vi "Concatenate PDF Standalone - V2.vi"(0 "New File name":path, 7 "PDF Files  to concatenate [ ]":T6[](array[typedef]), 11 "error in (no error)":errorcluster, 12 "PDF Details":T2, 13 "Permissions":T1={"User Password"="", "Owner Password"="", "Printing"=enum."Allow Printing", "Allow Modify Contents"=FALSE, "Allow Copy"=FALSE, "Allow Modify Annotations"=TRUE, "Allow Fill In "=TRUE, "Allow Screen Readers"=FALSE, "Allow Assembly"=FALSE}) -> (6 "Pages dimensions [ ] OUT":T3[](array[typedef]) {"Page Size" items=["Custom", "LETTER", "NOTE", "LEGAL", "TABLOID", "EXECUTIVE", "POSTCARD", "A0", "A1", "A2", "A3", "A4", "A5", "A6", "A7", "A8", "A9", "A10", "B0", "B1", "B2", "B3", "B4", "B5", "B6", "B7", "B8", "B9", "B10", "ARCH_E", "ARCH_D", "ARCH_C", "ARCH_B", "ARCH_A", "FLSA", "FLSE", "HALFLETTER", "_11X17", "ID_1", "ID_2", "ID_3", "LEDGER", "CROWN_QUARTO", "LARGE_CROWN_QUARTO", "DEMY_QUARTO", "ROYAL_QUARTO", "CROWN_OCTAVO", "LARGE_CROWN_OCTAVO", "DEMY_OCTAVO", "ROYAL_OCTAVO", "SMALL_PAPERBACK", "PENGUIN_SMALL_PAPERBACK", "PENGUIN_LARGE_PAPERBACK"]}, 15 "error out":errorcluster)   [LabVIEW 2019, in "Exaprom PDF.lvlib"]
doc: "Standalone.\n\nVersion 1.0\nDeveloped by Jean-Marc Simard\nCopyright © 2012, Exaprom Inc.\nAll rights reserved.\nLicense: BSD\n\nWith iTextSharp Library\n(http://itextsharp.sourceforge.net)"
uses:
  Controls/Concatenate Controls/PDF file to concatenate.ctl
  Controls/Page Controls/Page dimensions.ctl
  Controls/Page Controls/Page Orientation.ctl
  Controls/Initialization Controls/PDF Details.ctl
  Controls/Initialization Controls/File Permission Parameters.ctl
  Controls/General Controls/Create or close.ctl
  Controls/Concatenate Controls/PDF File and position.ctl
  Controls/Concatenate Controls/PDF file source.ctl
  Exaprom PDF.lvlib
  Controls/Page Controls/Page size.ctl
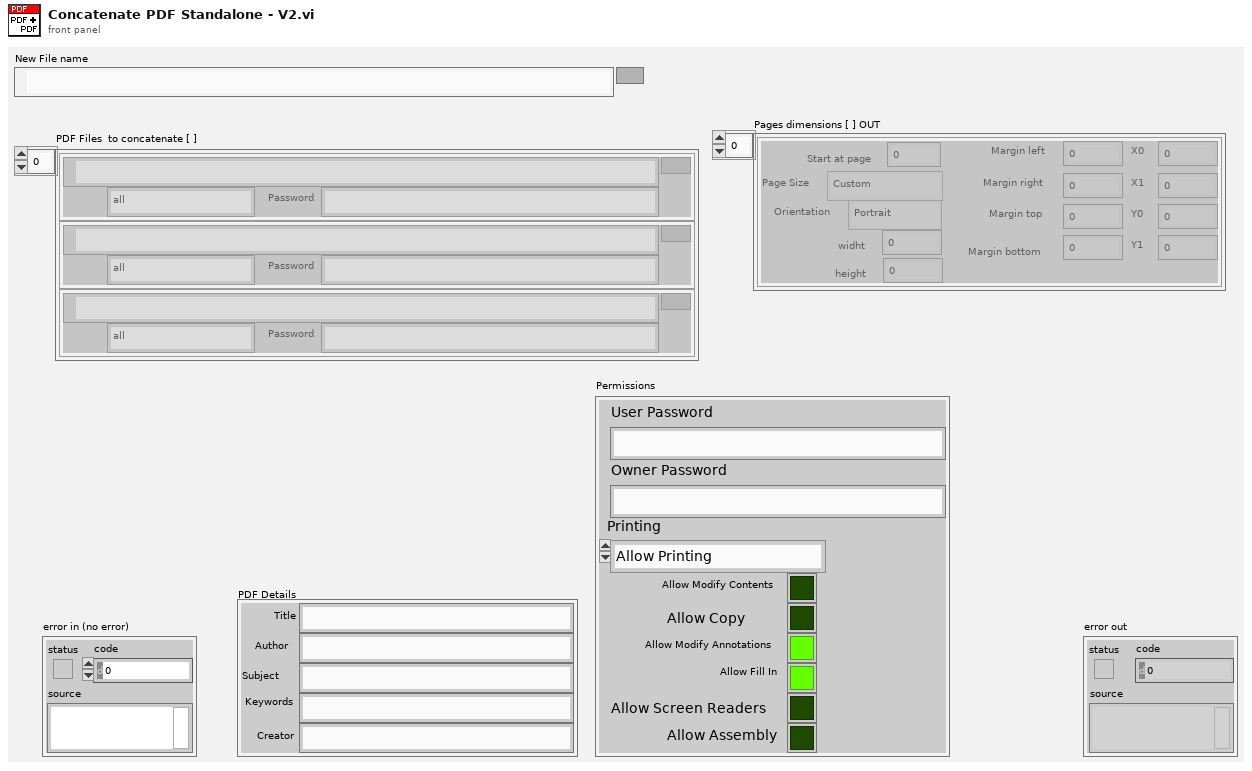
[diagram p1: front panel]
types:
  T1 = typedef "Exaprom PDF.lvlib/File Permission Parameters.ctl" = cluster{"User Password":string, "Owner Password":string, "Printing":enum16{"Allow Printing", "Allow Degraded Printing", "Don't Allow Printing"}, "Allow Modify Contents":bool, "Allow Copy":bool, "Allow Modify Annotations":bool, "Allow Fill In ":bool, "Allow Screen Readers":bool, "Allow Assembly":bool}
  T2 = typedef "Exaprom PDF.lvlib/PDF Details.ctl" = cluster{"Title":string, "Author":string, "Subject":string, "Keywords":string, "Creator":string}
  T3 = typedef "Exaprom PDF.lvlib/Page dimensions.ctl" = cluster{"Start at page":i32, "Page Size":T4, "Orientation":T5, "widht":sgl, "height":sgl, "Margin left":sgl, "Margin right":sgl, "Margin top":sgl, "Margin bottom":sgl, "X0":sgl, "X1":sgl, "Y0":sgl, "Y1":sgl}
  T4 = typedef "Exaprom PDF.lvlib/Page size.ctl" = i32
  T5 = typedef "Exaprom PDF.lvlib/Page Orientation.ctl" = enum16{"Portrait", "Landscape"}
  T6 = typedef "Exaprom PDF.lvlib/PDF file to concatenate.ctl" = cluster{"Path":path, "Pages":string, "Password":string}
  T7 = typedef "Exaprom PDF.lvlib/Create or close.ctl" = enum16{"Create", "Close"}
  T8 = typedef "Exaprom PDF.lvlib/PDF File and position.ctl" = cluster{"Path":path, "Pages":string, "Source":T9, "Start at page old":i32, "Start at page new":i32, "Owner password":string}
  T9 = typedef "Exaprom PDF.lvlib/PDF file source.ctl" = enum16{"PDF Report", "File to add"}
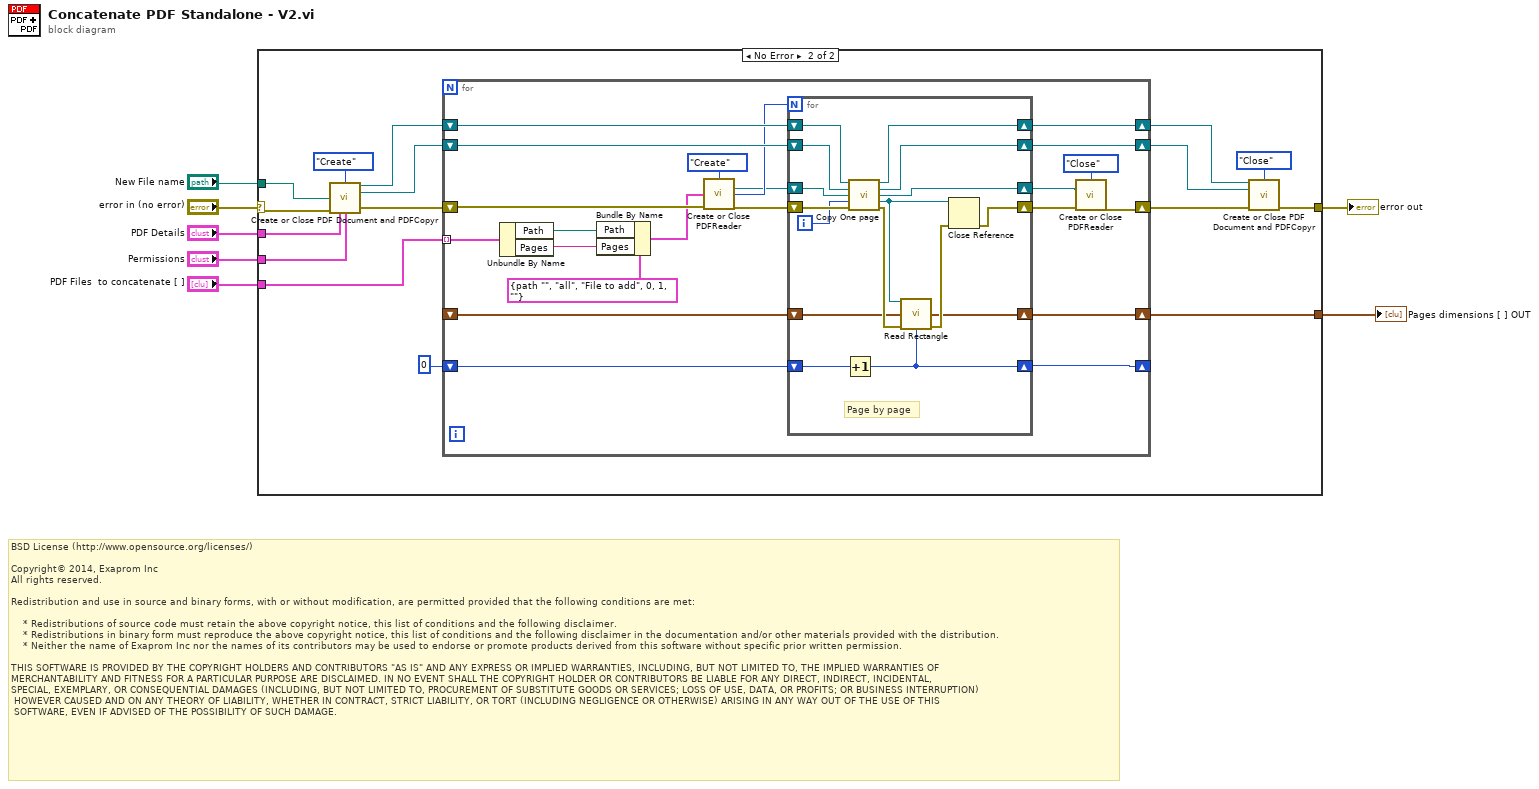
[diagram p0: block diagram]
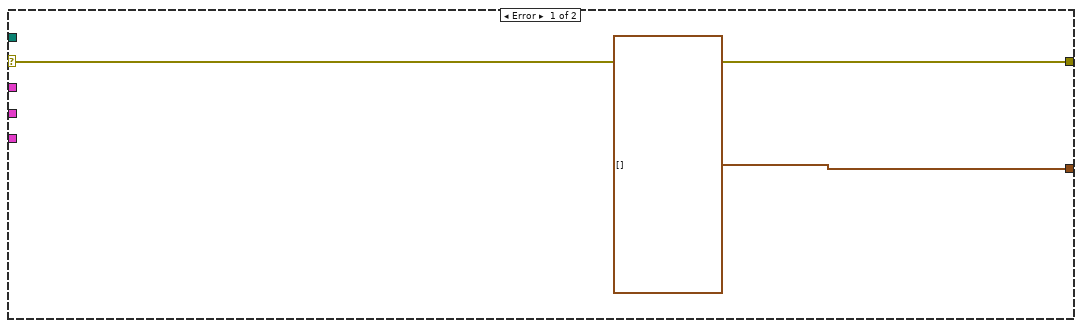
[diagram p2: hidden frame]
diagram:
  # "BSD License (http://www.opensource.org/licenses/)\n\nCopyright© 2014, Exaprom Inc\nAll rights reserved.\n\nRedistribution and use in source and binary forms, with or without modification, are permitted provided that the following conditions are met:\n\n    * Redistributions of source code must retain the above copyright notice, this list of conditions and the following disclaimer.\n    * Redistributions in binary form must reproduce the above copyright notice, this list of conditions and the following disclaimer in the documentation and/or other materials provided with the distribution.\n    * Neither the name of Exaprom Inc nor the names of its contributors may be used to endorse or promote products derived from this software without specific prior written permission.\n\nTHIS SOFTWARE IS PROVIDED BY THE COPYRIGHT HOLDERS AND CONTRIBUTORS \"AS IS\" AND ANY EXPRESS OR IMPLIED WARRANTIES, INCLUDING, BUT NOT LIMITED TO, THE IMPLIED WARRANTIES OF \nMERCHANTABILITY AND FITNESS FOR A PARTICULAR PURPOSE ARE DISCLAIMED. IN NO EVENT SHALL THE COPYRIGHT HOLDER OR CONTRIBUTORS BE LIABLE FOR ANY DIRECT, INDIRECT, INCIDENTAL,\nSPECIAL, EXEMPLARY, OR CONSEQUENTIAL DAMAGES (INCLUDING, BUT NOT LIMITED TO, PROCUREMENT OF SUBSTITUTE GOODS OR SERVICES; LOSS OF USE, DATA, OR PROFITS; OR BUSINESS INTERRUPTION)\n HOWEVER CAUSED AND ON ANY THEORY OF LIABILITY, WHETHER IN CONTRACT, STRICT LIABILITY, OR TORT (INCLUDING NEGLIGENCE OR OTHERWISE) ARISING IN ANY WAY OUT OF THE USE OF THIS\n SOFTWARE, EVEN IF ADVISED OF THE POSSIBILITY OF SUCH DAMAGE."
  n1 = case shown="No Error" "error in (no error)" {
    selector: "error in (no error)" -> [w9 w23]
    tunnel: [w9 w17] -> w7
    tunnel: "New File name" -> [_ w20]
    tunnel: "PDF Files  to concatenate [ ]" -> [_ w25]
    tunnel: [T3[] [] ("Pages dimensions [ ] OUT") w12] -> w3
    tunnel: "PDF Details" -> [_ w11]
    tunnel: "Permissions" -> [_ w10]
    frame Error {
    }
    frame No Error {
      n2 = call "Create or Close PDF Document and PDFCopyr.vi"("Action"=Create_or_close."Create", "File name"=w20, "error in (no error)"=w23, "PDF Details"=w11, "Permissions"=w10) -> ("PDF Copy OUT"=w22:refnum<k24>, "PDF Document OUT"=w21:refnum<k24>, "error out"=w24:errorcluster)  [unwired: 8 in]
      n3 = for {
        tunnel: w25 -> [w34] mode=indexing
        shift-right: [w45] -> w15
        shift-left: w21 -> [w47]
        shift-right: [w37] -> w18
        shift-left: w24 -> [w42]
        shift-right: [w44] -> w16
        shift-left: w22 -> [w46]
        shift-right: [w29] -> w12
        shift-left: _ -> [w28]
        shift-right: [w26] -> _
        shift-left: 0 -> [w27]
        n4 = Unbundle By Name(w34) -> ("Path"=w32:path, "Pages"=w31:string)
        n5 = Bundle By Name(cluster=T8 {"Path"=path "", "Pages"="all", "Source"=enum."File to add", "Start at page old"=0, "Start at page new"=1, "Owner password"=""} ("PDF File and position"), "Path"=w32, "Pages"=w31) -> (w30:T8)
        n6 = call "Create or Close PDFReader.vi"("Action"=Create_or_close."Create", "PDF File and position"=w30, "error in (no error)"=w42) -> ("PdfReader OUT"=w40:refnum<k24>, "NumberOfPages"=w41:i32, "error out"=w43:errorcluster)  [unwired: 8 in, 2 out]
        n7 = for {
          N: w41 -> [_]
          shift-right: [w56] -> w45
          shift-left: w47 -> [w60]
          shift-right: [w55] -> w38
          shift-left: w40 -> [w61]
          shift-right: [w51] -> w39
          shift-left: w43 -> [w62]
          shift-right: [w57] -> w44
          shift-left: w46 -> [w59]
          shift-right: [w53] -> w29
          shift-left: w28 -> [w52]
          shift-right: [w48] -> w26
          shift-left: w27 -> [w49]
          i -> [w58]
          # "Page by page"
          n8 = Increment(x=w49) -> (x+1=w48:i32)
          n9 = call "Copy One page.vi"("PDFCopy IN"=w59, "PDF Document IN"=w60, "PdfReader IN"=w61, "index"=w58, "error in (no error)"=w62) -> ("PDFCopy OUT"=w57:refnum<k24>, "PDF Document OUT"=w56:refnum<k24>, "PdfReader OUT"=w55:refnum<k24>, "GetPageSizeWithRotation"=w50:refnum<k24>, "error out"=w54:errorcluster)  [unwired: 6 in]
          n10 = call "Read Rectangle.vi"("GetPageSizeWithRotation"=w50, "Pages dimensions [ ] IN"=w52, "error in (no error)"=w54, "Start at page"=w48) -> ("Pages dimensions [ ] OUT"=w53:T3[], "error out"=w63:errorcluster)  [unwired: 10 in]
          n11 = Close Reference(reference=w50, error in (no error)=w63) -> (error out=w51:errorcluster)
        }
        n12 = call "Create or Close PDFReader.vi"("Action"=Create_or_close."Close", "PdfReader IN"=w38, "error in (no error)"=w39) -> ("error out"=w37:errorcluster)  [unwired: 8 in, 4 out]
      }
      n13 = call "Create or Close PDF Document and PDFCopyr.vi"("PDF Copy IN"=w16, "Action"=Create_or_close."Close", "PDF Document IN"=w15, "error in (no error)"=w18) -> ("error out"=w17:errorcluster)  [unwired: 9 in, 2 out]
    }
  }
  "error out" <- w7
  "Pages dimensions [ ] OUT" <- w3
